vi "Has Next.vi"(8 "error in (no error)":errorcluster, 11 "Double Scanner.lvclass in":refnum<class "Double Scanner.lvclass">) -> (0 "error out":errorcluster, 2 "Again?":bool, 3 "Double Scanner.lvclass out":refnum<class "Double Scanner.lvclass">)   [LabVIEW 2012, in "Double Scanner.lvclass"]
doc: "(Dynamic) Return TRUE if this Scanner has not yet completed all steps in its preconfigured Range."
uses:
  Double Scanner.lvclass
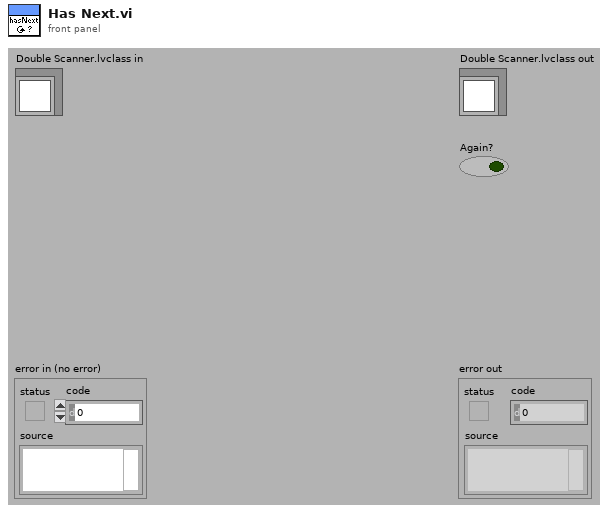
[diagram p1: front panel]
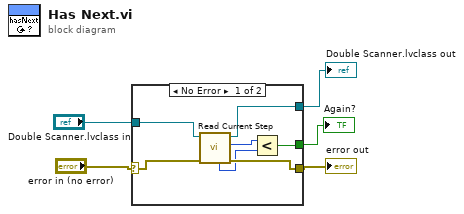
[diagram p0: block diagram]
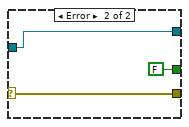
[diagram p2: hidden frame]
diagram:
  n1 = case shown="No Error" "error in (no error)" {
    selector: "error in (no error)" -> [w12 w15]
    tunnel: [w9 w15] -> w1
    tunnel: "Double Scanner.lvclass in" -> [w11 w14]
    tunnel: [w10 w14] -> w3
    tunnel: [w7 FALSE] -> w2
    frame No Error {
      n2 = call-dynamic "Read Current Step.vi"("error in (no error)"=w12, "Double Scanner in"=w11) -> ("error out"=w9:errorcluster, "Current step"=w8:u32, "Double Scanner out"=w10:refnum<class "Double Scanner.lvclass">, "Total steps"=w6:i32)  [unwired: 5 in, 1 out]
      n3 = Less?(x=w8, y=w6) -> (x < y?=w7:bool)
    }
    frame Error {
    }
  }
  "error out" <- w1
  "Double Scanner.lvclass out" <- w3
  "Again?" <- w2
